vi "Overhead_Factor.vi"(1 "Current Overhead Factor In":dbl format="%.1f", 2 "Sum of Ideal times (Sec)":dbl, 3 "Sum of Actual times (Sec)":dbl, 4 "Mode":T1) -> (0 "Current Overhead Factor":dbl format="%.1f")   [LabVIEW 2020]
uses:
  Controls/Overhead.ctl
panel:
  out "Ideal Register":dbl
  out "Actual Register":dbl
  out "Unclamped Factor":dbl format="%.2f"
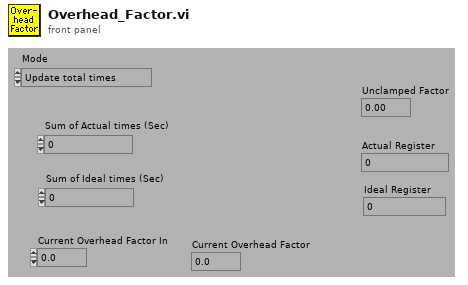
[diagram p1: front panel]
types:
  T1 = typedef "Overhead.ctl" = enum16{"Update total times", "Read Current Overhead", "Re Scale totals to 3 hrs", "Initialise totals to 3hr"}
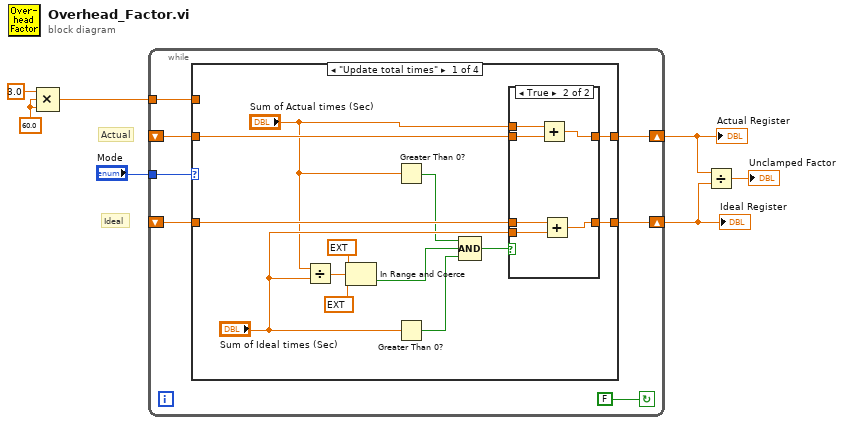
[diagram p0: block diagram]
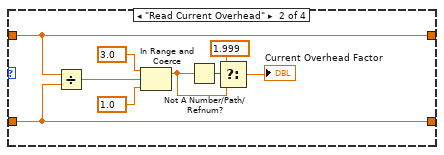
[diagram p3: hidden frame]
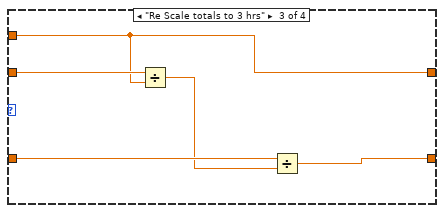
[diagram p4: hidden frame]
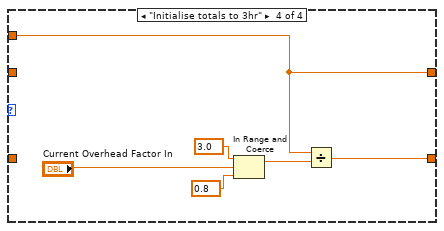
[diagram p5: hidden frame]
diagram:
  w2 = 60.0 ("value")
  # "Actual"
  # "Ideal"
  n1 = Compound Arithmetic op=MULTIPLY(3.0 ("value"), w2, w2) -> (w1:dbl)
  n2 = while {
    tunnel: w1 -> [w9]
    tunnel: "Mode" -> [w14]
    shift-left: _ -> [w11]
    shift-right: [w10] -> w5
    shift-left: _ -> [w13]
    shift-right: [w12] -> w6
    stop <- FALSE continue-if-true
    n3 = case shown="\"Update total times\"" w14 {
      tunnel: w13 -> [w27 w44 w49 _]
      tunnel: [w26 w44 w45 w51] -> w12
      tunnel: w11 -> [w25 w43 w48 _]
      tunnel: [w24 w43 w46 w52] -> w10
      tunnel: w9 -> [_ _ w45 w51]
      frame "Update total times" {
        n4 = Divide(x="Sum of Actual times (Sec)", y="Sum of Ideal times (Sec)") -> (x/y=w21:dbl)
        n5 = In Range and Coerce(upper limit=ext 4.0 ("hi"), x=w21, lower limit=ext 0.8 ("lo")) -> (In Range?=w16:bool)  [unwired: 1 out]
        n6 = Greater Than 0?(x="Sum of Actual times (Sec)") -> (x > 0?=w17:bool)
        n7 = Greater Than 0?(x="Sum of Ideal times (Sec)") -> (x > 0?=w18:bool)
        n8 = Compound Arithmetic op=AND(w17, w16, w18) -> (w15:bool)
        n9 = case shown="True" w15 {
          tunnel: "Sum of Actual times (Sec)" -> [_ w35]
          tunnel: w27 -> [w29 w34]
          tunnel: [w29 w33] -> w26
          tunnel: w25 -> [w28 w32]
          tunnel: [w28 w31] -> w24
          tunnel: "Sum of Ideal times (Sec)" -> [_ w30]
          frame False {
          }
          frame True {
            n10 = Add(x=w35, y=w34) -> (x+y=w33:dbl)
            n11 = Add(x=w32, y=w30) -> (x+y=w31:dbl)
          }
        }
      }
      frame "Read Current Overhead" {
        n12 = Divide(x=w44, y=w43) -> (x/y=w40:dbl)
        n13 = In Range and Coerce(upper limit=3.0 ("Max"), x=w40, lower limit=1.0 ("Min")) -> (coerced(x)=w37:dbl)  [unwired: 1 out]
        n14 = Not A Number/Path/Refnum?(number/path/refnum=w37) -> (NaN/Path/Refnum?=w39:bool)
        n15 = Select(t=1.999, s=w39, f=w37) -> (s? t:f=→"Current Overhead Factor":dbl)
      }
      frame "Re Scale totals to 3 hrs" {
        n16 = Divide(x=w49, y=w45) -> (x/y=w47:dbl)
        n17 = Divide(x=w48, y=w47) -> (x/y=w46:dbl)
      }
      frame "Initialise totals to 3hr" {
        n18 = In Range and Coerce(upper limit=3.0 ("Max"), x="Current Overhead Factor In", lower limit=0.8 ("Min")) -> (coerced(x)=w50:dbl)  [unwired: 1 out]
        n19 = Divide(x=w51, y=w50) -> (x/y=w52:dbl)
      }
    }
  }
  "Actual Register" <- w6
  "Ideal Register" <- w5
  n20 = Divide(x=w6, y=w5) -> (x/y=→"Unclamped Factor":dbl)
